vi "Mod_OFDM_Set_Ofdm_Symbol.vi"(0 "Configuration out":variant, 2 "OFDM PARAMETERS":T6={"# of Sub Carrier"=64, "Length Of Cylic Prefix"=16}, 7 "Current OFDM Symbol":string, 11 "error in":errorcluster, 12 "Configure OFDM\nSymbol Settings":T7) -> (4 "Configuration out":variant, 15 "error out":errorcluster)   [LabVIEW 2010]
uses:
  Controls(Type_DEf)/Attribute Data Types.ctl
  Controls(Type_DEf)/Configure Pulse Shaping.ctl
  Controls(Type_DEf)/Pool of Modulator Control.ctl
  Controls(Type_DEf)/Pool of Data Source Control.ctl
  Controls(Type_DEf)/Attribute Names.ctl
panel:
  in  "Attribute Data Types":T1={"Pulse Shaping"={"System Filter"={"TX Filter"=enum."none", "Alpha"=0.0, "filter length"=0}, "Modulation system parameters"={"samples per symbol (16)"=0}, "symbol rate (Hz)"=0.0}, "FRAME Table"=[], "OFDM Frame"=[], "Sub Carrier Selection"={"Sub Carrier Selection"=array[10000 elements], "OFDM Parameters"={"# of Sub Carrier"=0, "Length Of Cylic Prefix"=0}}, "Symbol Table"=[], "Symbol Pool"=[], "Pool of Modulators"=[], "Pool of Data Sources"=[], "Atribute Names"={"Data Source Pool"="Data Source Pool ", "Modulator Source Pool"="Modulator Source Pool ", "OFDM SYMBOL POOL"="OFDM SYMBOL POOL", "Symbol Table"="Symbol Table", "Sub Carrier Selection"="Sub Carrier Selection", "OFDM Frame"="OFDM Frame", "FRAME Table"="FRAME Table", "Pulse Shaping"="Pulse Shaping"}} {"Pool of Data Sources"."Register Initial State" format="%08x"; "Pulse Shaping"."symbol rate (Hz)" min=1.0 step=1.0 format="%.2p"; "Pulse Shaping"."Modulation system parameters"."samples per symbol (16)" step=2; "Pulse Shaping"."System Filter"."Alpha" min=0.0 max=1.0 step=0.05 format="%.2f"}
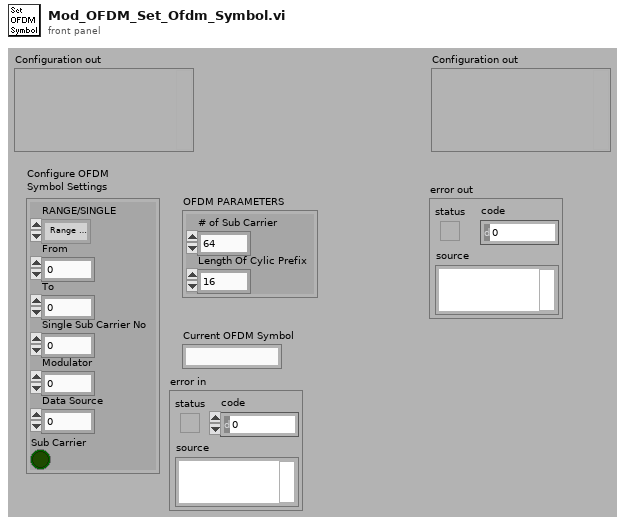
[diagram p1: front panel]
types:
  T1 = typedef "Attribute Data Types.ctl" = cluster{"Pulse Shaping":T2, "FRAME Table":string[][], "OFDM Frame":cluster{"Symbol Name":string, "# of Symbols":i32}[], "Sub Carrier Selection":cluster{"Sub Carrier Selection":cluster{"Sub Carrier":bool, "Data Source":u16, "Modulator":u16}[], "OFDM Parameters":cluster{"# of Sub Carrier":i32, "Length Of Cylic Prefix":i32}}, "Symbol Table":string[][], "Symbol Pool":string[], "Pool of Modulators":T3, "Pool of Data Sources":T4, "Atribute Names":T5}
  T2 = typedef "Configure Pulse Shaping.ctl" = cluster{"System Filter":cluster{"TX Filter":enum16{"none", "Raised Cosine", "Root Raised Cos"}, "Alpha":dbl, "filter length":i32}, "Modulation system parameters":cluster{"samples per symbol (16)":u32}, "symbol rate (Hz)":dbl}
  T3 = typedef "Pool of Modulator Control.ctl" = cluster{"M-QAM":enum16{"4", "16", "64", "256"}, "M-PSK":enum16{"2", "4", "8", "16", "32", "64", "128", "256"}, "Type of Modulation":enum16{"PSK", "QAM"}, " PSK":cluster{"differential PSK":enum16{"disable", "enable"}, "PSK type":enum16{"normal", "shifted", "offset"}}}[]
  T4 = typedef "Pool of Data Source Control.ctl" = cluster{"mode (PN)":enum16{"PN", "pattern", "user"}, "PN sequence order (9)":i32, "Invert Output Bits":enum16{"No", "Yes"}, "Register Initial State ":u32, "User base bit pattern":i8[], "base bit pattern (00001111)":enum16{"0", "1", "01", "0011", "00001111"}, "Reset to Initial State":enum16{"Every OFDM Frame", "Every OFDM Symbol", "Every Sub Carrier"}}[]
  T5 = typedef "Attribute Names.ctl" = cluster{"Data Source Pool":string, "Modulator Source Pool":string, "OFDM SYMBOL POOL":string, "Symbol Table":string, "Sub Carrier Selection":string, "OFDM Frame":string, "FRAME Table":string, "Pulse Shaping":string}
  T6 = cluster{"# of Sub Carrier":i32, "Length Of Cylic Prefix":i32}
  T7 = cluster{"RANGE/SINGLE":enum32{" Range of sub carriers", "Single sub carrier   "}, "From":i32, "To":i32, "Single Sub Carrier No":i32, "Modulator":u16, "Data Source":u16, "Sub Carrier":bool}
  T8 = cluster{"Sub Carrier":bool, "Data Source":u16, "Modulator":u16}
  T9 = cluster{"Sub Carrier Selection":cluster{"Sub Carrier":bool, "Data Source":u16, "Modulator":u16}[], "OFDM Parameters":cluster{"# of Sub Carrier":i32, "Length Of Cylic Prefix":i32}}
  T10 = enum32{" Range of sub carriers", "Single sub carrier   "}
  T11 = cluster{"Sub Carrier":bool, "Data Source":u16, "Modulator":u16}[]
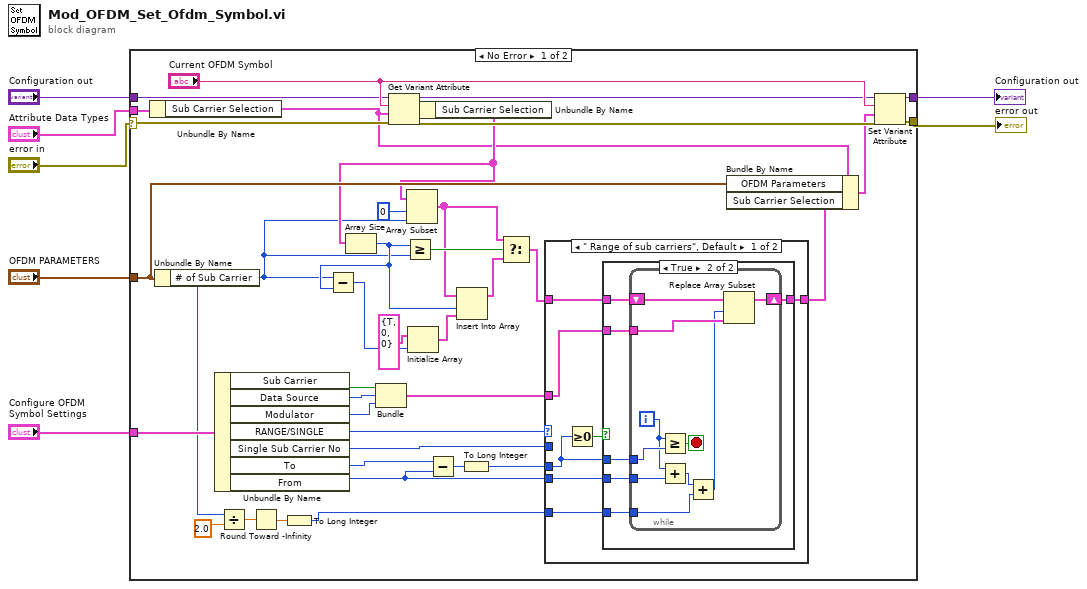
[diagram p0: block diagram]
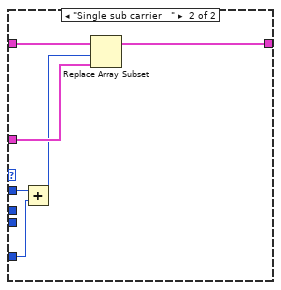
[diagram p3: hidden frame]
diagram:
  n1 = case shown="No Error" "error in" {
    selector: "error in" -> [w26 w77]
    tunnel: [w45 _] -> w7
    tunnel: "Configure OFDM\nSymbol Settings" -> [w37 _]
    tunnel: [w32 w77] -> w5
    tunnel: "Configuration out" -> [w25 _]
    tunnel: "OFDM PARAMETERS" -> [w24 _]
    tunnel: "Attribute Data Types" -> [w23 _]
    frame No Error {
      n2 = Unbundle By Name(w23) -> ("Sub Carrier Selection"=w8:T9)
      n3 = Unbundle By Name(w24) -> ("# of Sub Carrier"=w14:i32)
      n4 = Unbundle By Name(w37) -> ("Sub Carrier"=w33:bool, "Data Source"=w18:u16, "Modulator"=w17:u16, "RANGE/SINGLE"=w16:T10, "Single Sub Carrier No"=w34:i32, "To"=w35:i32, "From"=w36:i32)
      n5 = Divide(x=w14, y=2.0) -> (x/y=w12:dbl)
      n6 = Round Toward -Infinity(1:w12) -> (0:w11:dbl)
      n7 = To Long Integer(number=w11) -> (32bit integer=w10:i32)
      n8 = Bundle("Sub Carrier"=w33, "Data Source"=w18, "Modulator"=w17) -> (w46:T8)  [unwired: 1 in]
      n9 = Get Variant Attribute(Variant=w25, name="Current OFDM Symbol", default value (empty Variant)=w8, error in=w26) -> (duplicate Variant=w28:variant, value=w22:T9, error out=w27:errorcluster)  [unwired: 1 out]
      n10 = Unbundle By Name(w22) -> ("Sub Carrier Selection"=w21:T11)
      n11 = Array Size(array=w21) -> (size(s)=w15:i32)
      n12 = Subtract(x=w14, y=w15) -> (x-y=w38:i32)
      n13 = Greater Or Equal?(x=w15, y=w14) -> (x >= y?=w44:bool)
      n14 = Array Subset(array=w21, index=0, length=w14) -> (w42:T11)
      n15 = Initialize Array(T8 {"Sub Carrier"=TRUE, "Data Source"=0, "Modulator"=0} ("output cluster"), w38) -> (w31:T11)
      n16 = Subtract(x=w35, y=w36) -> (x-y=w20:i32)
      n17 = Insert Into Array(array=w42, index=w15, new element=w31) -> (w41:T11)
      n18 = To Long Integer(number=w20) -> (32bit integer=w19:i32)
      n19 = Select(t=w42, s=w44, f=w41) -> (s? t:f=w40:T11)
      n20 = case shown="\" Range of sub carriers\", Default" w16 {
        tunnel: w34 -> [_ w73]
        tunnel: w36 -> [w53 _]
        tunnel: w19 -> [w48 _]
        tunnel: w40 -> [w52 w76]
        tunnel: w46 -> [w50 w75]
        tunnel: [w51 w74] -> w30
        tunnel: w10 -> [w47 w72]
        frame " Range of sub carriers", Default {
          n21 = Greater Or Equal To 0?(x=w48) -> (x >= 0?=w49:bool)
          n22 = case shown="True" w49 {
            tunnel: w53 -> [_ w60]
            tunnel: w48 -> [_ w59]
            tunnel: w52 -> [w54 w58]
            tunnel: [w54 w57] -> w51
            tunnel: w50 -> [_ w56]
            tunnel: w47 -> [_ w55]
            frame False {
            }
            frame True {
              n23 = while {
                tunnel: w60 -> [w68]
                tunnel: w59 -> [w70]
                shift-right: [w65] -> w57
                shift-left: w58 -> [w66]
                tunnel: w56 -> [w64]
                tunnel: w55 -> [w62]
                i -> [w67]
                stop <- w69 stop-if-true
                n24 = Greater Or Equal?(x=w67, y=w70) -> (x >= y?=w69:bool)
                n25 = Add(x=w67, y=w68) -> (x+y=w63:i32)
                n26 = Add(x=w63, y=w62) -> (x+y=w61:i32)
                n27 = Replace Array Subset(array=w66, new element=w64, index=w61) -> (w65:T11)
              }
            }
          }
        }
        frame "Single sub carrier   " {
          n28 = Add(x=w73, y=w72) -> (x+y=w71:i32)
          n29 = Replace Array Subset(array=w76, new element=w75, index=w71) -> (w74:T11)
        }
      }
      n30 = Bundle By Name(cluster=w8, "OFDM Parameters"=w24, "Sub Carrier Selection"=w30) -> (w9:T9)
      n31 = Set Variant Attribute(Variant=w28, name="Current OFDM Symbol", value=w9, error in=w27) -> (Variant out=w45:variant, error out=w32:errorcluster)  [unwired: 1 out]
    }
    frame Error {
    }
  }
  "error out" <- w5
  "Configuration out" <- w7
